vi "slave diagnostic to string.vi"(11 "slave diagnostics":T1[](array[typedef])) -> (3 "data string":string)   [LabVIEW 2013, in "Profibus Module configuration.lvclass"]
uses:
  Profibus Module configuration.lvclass
  slave diagnostic configuration.ctl
  <vilib>/NI/Tag Bus Module Framework/channel/TBM channel.lvclass
  error throw specification.ctl
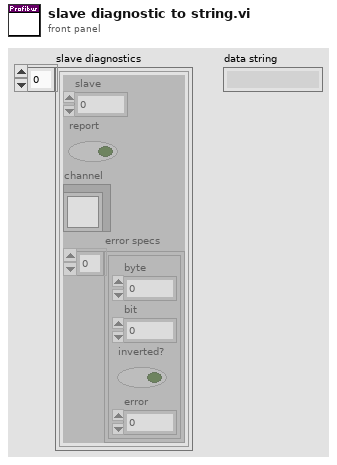
[diagram p1: front panel]
types:
  T1 = typedef "Profibus Module configuration.lvclass/slave diagnostic configuration.ctl" = cluster{"slave":i8, "report":bool, "channel":refnum<class "TBM channel.lvclass">, "error specs":T2[]}
  T2 = typedef "Profibus Module configuration.lvclass/error throw specification.ctl" = cluster{"byte":i32, "bit":i32, "inverted?":bool, "error":i32}
  T3 = cluster{"slave":i8, "identifier":string, "channel data":string, "error specs":T2[]}
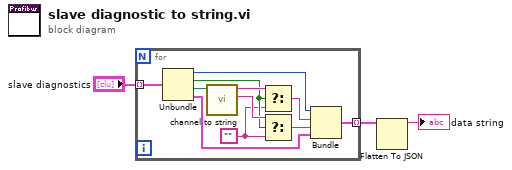
[diagram p0: block diagram]
diagram:
  n1 = for {
    tunnel: "slave diagnostics" -> [w14] mode=indexing
    tunnel: [w10] -> w2 mode=indexing
    w4 = ""
    n2 = Unbundle(w14) -> ("slave"=w13:i8, "report"=w7:bool, "channel"=w11:refnum<class "TBM channel.lvclass">, "error specs"=w12:T2[])
    n3 = call <vilib>:"channel to string.vi"("channel in"=w11) -> ("channel data"=w8:string, "identifier"=w9:string)  [unwired: 9 in]
    n4 = Select(t=w9, s=w7, f=w4) -> (s? t:f=w5:string)
    n5 = Select(t=w8, s=w7, f=w4) -> (s? t:f=w6:string)
    n6 = Bundle("slave"=w13, "identifier"=w5, "channel data"=w6, "error specs"=w12) -> (w10:T3)  [unwired: 1 in]
  }
  n7 = Flatten To JSON(anything=w2) -> (JSON string=→"data string":string)  [unwired: 2 in, 1 out]
